vi "PH_Beckhoff_PP_Control.open Mercury PSDB Connection.vi"(0 "i ref in":refnum<vi>, 5 "error in":errorcluster) -> (14 "i ref out":refnum<vi>, 19 "error out":errorcluster)   [LabVIEW 2014, in "PH_Beckhoff_PP_Control.lvlib"]
doc: "This VI opens the connection to the PSDB to get the necessary IDs and opens the related DIM services."
uses:
  PH_Beckhoff_PP_Control.lvlib
  PH_PSDBWriter/PH_PSDBWriter.PHELIX-Subsystems.ctl
  PH_Beckhoff_Common/PH_Beckhoff_Common.former PSDB classes.ctl
  PH_PSDBWriter/PH_PSDBWriter.Data Status.ctl
  PH_PSDBWriter/PH_PSDBWriter.lvlib
  lib.lib/DimLVEvent/LVDimInterface/LVDimInterface.lvlib
  PH_Beckhoff_Common/PH_Beckhoff_Common.lvlib
  PH_Common/PH_Common.lvlib
panel:
  in  "PHELIX Subsysteme":T1 items=["Miscellaneous", "fs-Frontend", "ns-Frontend", "PreAmp", "MainAmp", "MAS", "COS", "Beamline", "Experiment Laserbay", "Experiment Laserlabor", "Experiment Z6", "Timing", "Pulsed Power"]
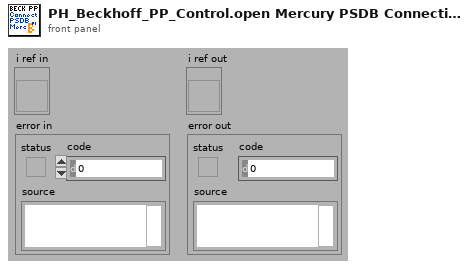
[diagram p1: front panel]
types:
  T1 = typedef "PH_PSDBWriter.lvlib/PH_PSDBWriter.PHELIX-Subsystems.ctl" = i32
  T2 = typedef "PH_Beckhoff_Common.lvlib/PH_Beckhoff_Common.former PSDB classes.ctl" = enum16{"PP Conductivity", "PP Mercury", "PA Chiller"}
  T3 = typedef "PH_Beckhoff_PP_Control.lvlib/PH_Beckhoff_PP_Control.i attribute.ctl" = cluster{"PP Conductivity Control":cluster{"PSDB":cluster{"Status Service ID":i32, "Instance ID":i32, "Data Status":T4, "Ref Status":refnum<vi>, "Error Code":i32}, "Status":cluster{"GUI Ref":refnum<vi>, "Status Service ID":i32, "Status":T5}, "DIs":cluster{"Device on":cluster{"GUI Ref":refnum<vi>, "# in Data":i32}, "Conductivity ok":cluster{"GUI Ref":refnum<vi>, "# in Data":i32}, "Temperature ok":cluster{"GUI Ref":refnum<vi>, "# in Data":i32}, "Alarm":cluster{"GUI Ref":refnum<vi>, "# in Data":i32}}, "PSDB Thread":cluster{"Ref":refnum<vi>, "Q-Ref":refnum<queue>}}, "PP Mercury Control":cluster{"PSDB":cluster{"Status Service ID":i32, "Instance ID":i32, "Data Status":T4, "Ref Status":refnum<vi>, "Error Code":i32}, "Status":cluster{"GUI Ref":refnum<vi>, "Status Service ID":i32, "Status":T5}, "on since:":cluster{"GUI Ref":refnum<vi>, "Service ID":i32, "Time":string}, "DIs":cluster{"Device on":cluster{"GUI Ref":refnum<vi>, "# in Data":i32}, "Alarm":cluster{"GUI Ref":refnum<vi>, "# in Data":i32}}, "AIs":cluster{"Concentration":cluster{"GUI Ref":refnum<vi>, "# in Data":i32}}, "PSDB Thread":cluster{"Ref":refnum<vi>, "Q-Ref":refnum<queue>}}, "PSDB":cluster{"Shot #":i32, "Subsystem":T1}, "PSDB Credentials":T6}
  T4 = typedef "PH_PSDBWriter.lvlib/PH_PSDBWriter.Data Status.ctl" = i16
  T5 = typedef "PH_StatusHandler.lvlib/PH_StatusHandler.Status.ctl" = i16
  T6 = typedef "PH_Common.lvlib/PH_Connection.PSDB Credentials.ctl" = cluster{"PW":string, "ID":string, "DS":string}
  T7 = cluster{"Instancename":string, "Classname":string}
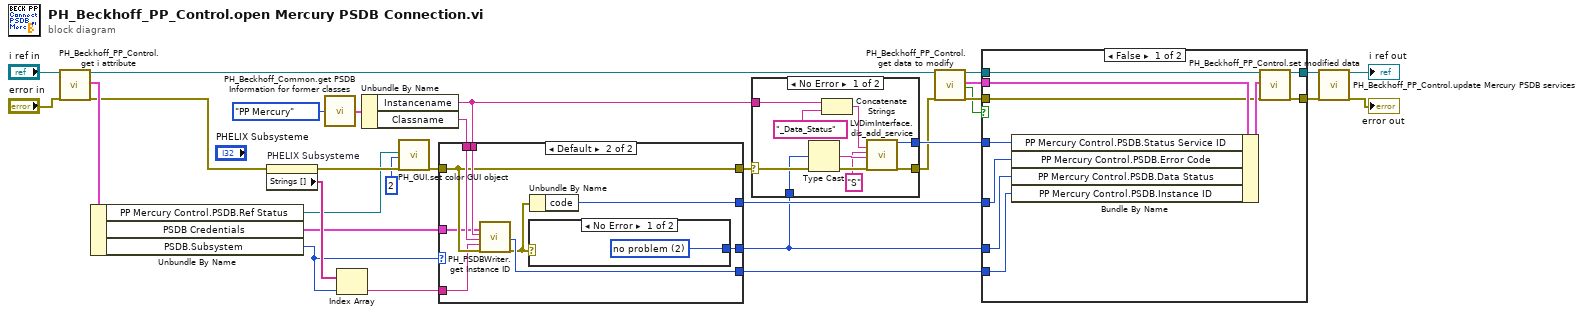
[diagram p0: block diagram]
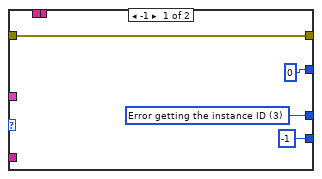
[diagram p2: hidden frame]
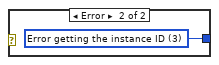
[diagram p3: hidden frame]
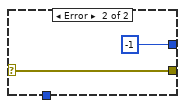
[diagram p4: hidden frame]
diagram:
  n1 = call "PH_Beckhoff_PP_Control.get i attribute.vi"("i ref in"="i ref in", "error in (no error)"="error in") -> ("i ref out"=w30:refnum<vi>, "i attribute"=w31:T3, "error out"=w28:errorcluster)  [unwired: 15 in]
  n2 = Unbundle By Name(w31) -> ("PP Mercury Control.PSDB.Ref Status"=w10:refnum<vi>, "PSDB Credentials"=w1:T6, "PSDB.Subsystem"=w21:T1)
  n3 = property on="PHELIX Subsysteme" class="Ring (strict)"(error in=w28) -> (error out=w22:errorcluster, "Strings []"=w24:string[])  [unwired: 1 in, 1 out]
  n4 = call "PH_Beckhoff_Common.get PSDB Information for former classes.vi"("PSDB Classes"=PH_Beckhoff_Common.former_PSDB_classes."PP Mercury") -> ("PSDB Information"=w17:T7)
  n5 = Index Array(array=w24, index=w21) -> (element=w23:string)
  n6 = Unbundle By Name(w17) -> ("Instancename"=w8:string, "Classname"=w7:string)
  n7 = call "PH_GUI.set color GUI object.vi"("GUI object Ref"=w10, "State"=2, "error in (no error)"=w22) -> ("error out"=w5:errorcluster)  [unwired: 16 in]
  n8 = case shown="Default" w21 {
    tunnel: [w35 w44] -> w19
    tunnel: [-1 ("instance_id") w39] -> w18
    tunnel: w5 -> [w33 w40]
    tunnel: [w33 w40] -> w9
    tunnel: [0 ("code") w43] -> w20
    tunnel: w23 -> [_ w38]
    tunnel: w8 -> [_ w41]
    tunnel: w7 -> [_ w42]
    tunnel: w1 -> [_ w36]
    frame -1 {
      w35 = T4 3 items=["no info", "no Data collection", "no problem", "Error getting the instance ID", "Error writing Data to data base", "Error concerning the subsystem"] ("Metadata.Data Status")
    }
    frame Default {
      n9 = call "PH_PSDBWriter.get Instance ID.vi"("PSDB Credentials"=w36, "Instace Name"=w41, "Class"=w42, "Subsystem"=w38, "error in"=w40) -> ("instance_id"=w39:i32, "error out"=w37:errorcluster)  [unwired: 13 in]
      n10 = case shown="No Error" w37 {
        tunnel: [w45 w46] -> w44
        frame No Error {
          w45 = T4 2 items=["no info", "no Data collection", "no problem", "Error getting the instance ID", "Error writing Data to data base"] ("Metadata.Data Status")
        }
        frame Error {
          w46 = T4 3 items=["no info", "no Data collection", "no problem", "Error getting the instance ID", "Error writing Data to data base"] ("Metadata.Data Status")
        }
      }
      n11 = Unbundle By Name(w37) -> ("code"=w43:i32)
    }
  }
  n12 = case shown="No Error" w9 {
    selector: w9 -> [w53 w57]
    tunnel: [w55 -1 ("my_serviceID")] -> w25
    tunnel: [w54 w57] -> w14
    tunnel: w8 -> [w48 _]
    tunnel: w19 -> [w47 _]
    frame No Error {
      n13 = Type Cast(x=w47) -> (*(type *) &x=w52:string)  [unwired: 1 in]
      n14 = Concatenate Strings(w48, "_Data_Status" ("string")) -> (w50:string)
      n15 = call "LVDimInterface.dis_add_service.vi"("serviceName"=w50, "typeDescriptor"="S", "data"=w52, "error in (no error)"=w53) -> ("my_serviceID"=w55:i32, "error out"=w54:errorcluster)  [unwired: 14 in]
    }
    frame Error {
    }
  }
  n16 = call "PH_Beckhoff_PP_Control.get data to modify.vi"("i ref in"=w30, "error in (no error)"=w14) -> ("i ref out"=w16:refnum<vi>, "i attribute"=w15:T3, "timed out"=w12:bool, "error out"=w13:errorcluster)  [unwired: 14 in]
  n17 = case shown="False" w12 {
    tunnel: [w67 w69] -> w3
    tunnel: [w66 w68] -> w26
    tunnel: w25 -> [w61 _]
    tunnel: w20 -> [w60 _]
    tunnel: w19 -> [w59 _]
    tunnel: w18 -> [w58 _]
    tunnel: w16 -> [w64 w69]
    tunnel: w15 -> [w63 _]
    tunnel: w13 -> [w62 w68]
    frame False {
      n18 = Bundle By Name(cluster=w63, "PP Mercury Control.PSDB.Status Service ID"=w61, "PP Mercury Control.PSDB.Error Code"=w60, "PP Mercury Control.PSDB.Data Status"=w59, "PP Mercury Control.PSDB.Instance ID"=w58) -> (w65:T3)
      n19 = call "PH_Beckhoff_PP_Control.set modified data.vi"("i ref in"=w64, "i attribute"=w65, "error in (no error)"=w62) -> ("i ref out"=w67:refnum<vi>, "error out"=w66:errorcluster)  [unwired: 15 in]
    }
    frame True {
    }
  }
  n20 = call "PH_Beckhoff_PP_Control.update Mercury PSDB services.vi"("i ref in"=w3, "error in"=w26) -> ("i ref out"=→"i ref out":refnum<vi>, "error out"=→"error out":errorcluster)  [unwired: 16 in]
